vi "Write to Database.vi"(0 "File Data Manager in":refnum<class "File Data Manager.lvclass">, 5 "DB to Write":T1[](array[typedef]), 11 "error in (no error)":errorcluster) -> (4 "File Data Manager out":refnum<class "File Data Manager.lvclass">, 15 "error out":errorcluster)   [LabVIEW 2023, in "File Data Manager.lvlib" / "File Data Manager.lvclass"]
uses:
  File Data Manager.lvclass
  File Data Manager.lvclass/File Data Manager.ctl
  Database Selection.ctl
  Central Data Manager/Central Data Manager/Central Data Manager.lvclass
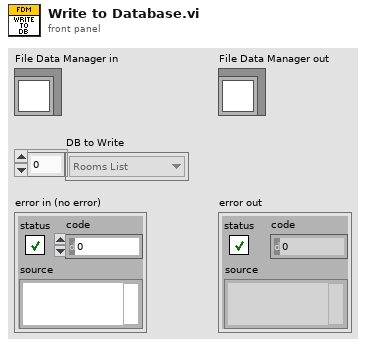
[diagram p1: front panel]
types:
  T1 = typedef "Central Data Manager.lvlib/Central Data Manager.lvclass/Database Selection.ctl" = enum16{"Rooms List", "Guests History"}
  T2 = typedef "Central Data Manager.lvlib/Central Data Manager.lvclass/Guest Details.ctl" = cluster{"Contact Number":string, "Primary Guest Name":string}
  T3 = typedef "Central Data Manager.lvlib/Central Data Manager.lvclass/Room Details.ctl" = cluster{"Room No":string, "Room Size":string, "Room Occupancy Status":T4, "Guest Details":T2, "Occupancy Count (Adult)":u32, "Occupancy Count (Children)":u32, "Check-in Time":timestamp, "Check-out Time":timestamp}
  T4 = typedef "Central Data Manager.lvlib/Central Data Manager.lvclass/Room Occupancy Status.ctl" = enum16{"Not Occupied", "Occupied", "Under Maintainance", "Not Servicable"}
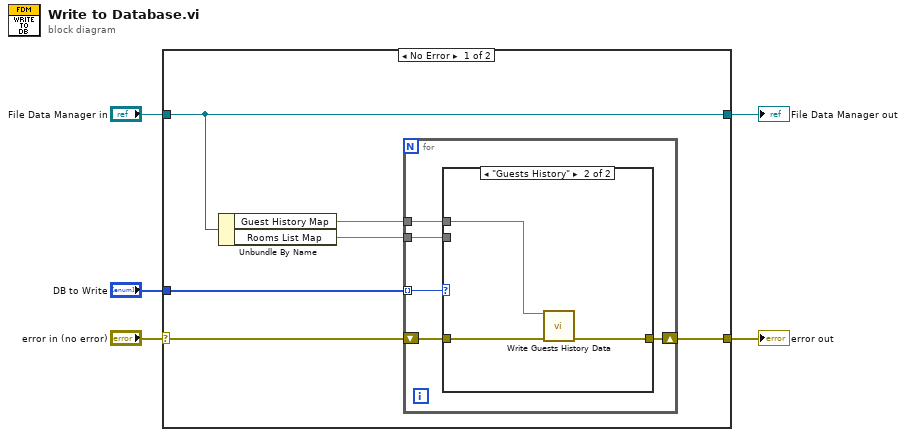
[diagram p0: block diagram]
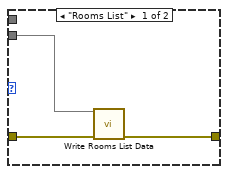
[diagram p2: hidden frame]
diagram:
  n1 = case shown="No Error" "error in (no error)" {
    selector: "error in (no error)" -> [w7 w24]
    tunnel: [w10 w24] -> w4
    tunnel: [w11 w23] -> w2
    tunnel: "File Data Manager in" -> [w11 w23]
    tunnel: "DB to Write" -> [w6 _]
    frame No Error {
      n2 = Unbundle By Name(w11) -> ("Guest History Map"=w9:map{string, T2}, "Rooms List Map"=w8:map{string, T3})
      n3 = for {
        tunnel: w9 -> [w15]
        tunnel: w8 -> [w14]
        tunnel: w6 -> [w12] mode=indexing
        shift-right: [w16] -> w10
        shift-left: w7 -> [w13]
        n4 = case shown="\"Guests History\"" w12 {
          tunnel: [w17 w22] -> w16
          tunnel: w15 -> [_ w21]
          tunnel: w14 -> [w19 _]
          tunnel: w13 -> [w18 w20]
          frame "Rooms List" {
            n5 = call "Write Rooms List Data.vi"("Rooms List Map"=w19, "error in (no error)"=w18) -> ("error out"=w17:errorcluster)  [unwired: 13 in]
          }
          frame "Guests History" {
            n6 = call "Write Guests History Data.vi"("Guest History Map"=w21, "error in (no error)"=w20) -> ("error out"=w22:errorcluster)  [unwired: 13 in]
          }
        }
      }
    }
    frame Error {
    }
  }
  "error out" <- w4
  "File Data Manager out" <- w2
